vi "FTP Move_Status_Errors.vi"(6 "remote port (21)":u16=21, 8 "error in (no error)":errorcluster, 9 "Dir of file to FTP":path, 10 "FTP input cluster":T1 {"FTP Timeout (S)" min=0 max=300 step=1}, 11 "File to Move":string) -> (1 "concatenated string of Error":string, 3 "FTP completed (true = good)":bool)   [LabVIEW 2011]
uses:
  Controls/FTP Credintials.ctl
  <vilib>/addons/internet/NI_InternetTK_FTP_VIs.lvlib
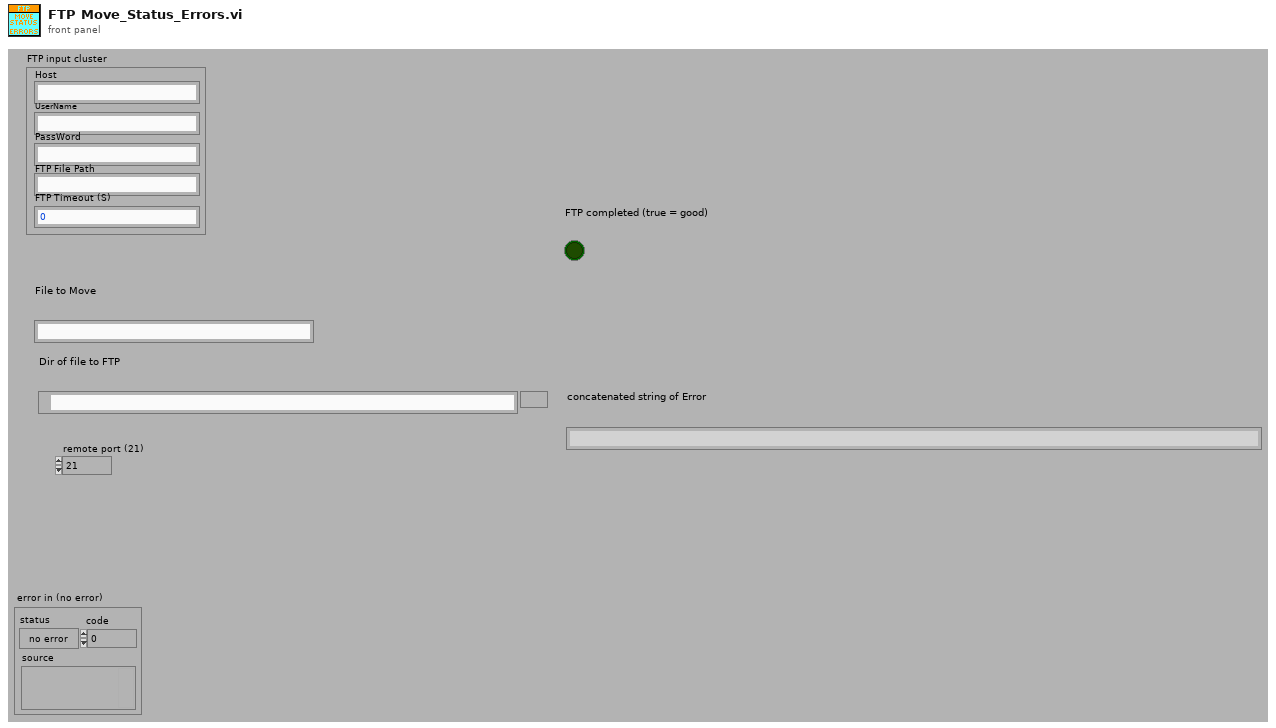
[diagram p1: front panel]
types:
  T1 = typedef "FTP Credintials.ctl" = cluster{"Host":string, "UserName":string, "PassWord":string, "FTP File Path":string, "FTP Timeout (S)":i32, "Active or Passive":bool, "ASCII or Binary":bool}
  T2 = typedef "FTP Session.ctl" = refnum<k1>
  T3 = cluster{string, "appended path":path, "ASCII or Binary":bool, string}
  T4 = cluster{string, "appended path":path, "ASCII or Binary":bool, string}[]
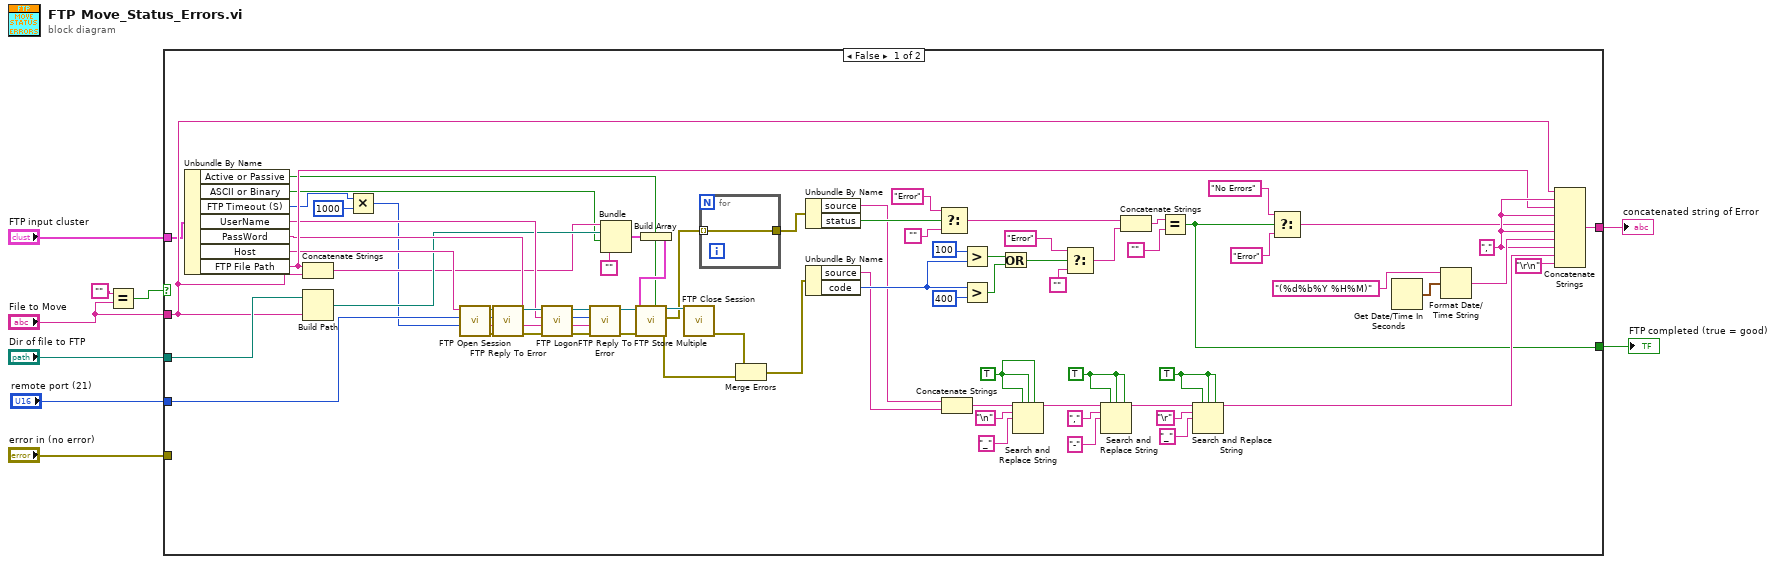
[diagram p0: block diagram]
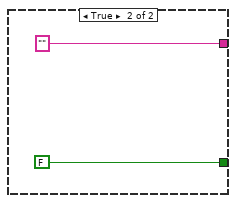
[diagram p2: hidden frame]
diagram:
  n1 = Equal?(x="", y="File to Move") -> (x = y?=w3:bool)
  n2 = case shown="False" w3 {
    tunnel: "Dir of file to FTP" -> [w69 _]
    tunnel: [w68 ""] -> w8
    tunnel: "File to Move" -> [w67 _]
    tunnel: "FTP input cluster" -> [w66 _]
    tunnel: [w12 FALSE] -> w7
    tunnel: "error in (no error)" -> [_ _]
    tunnel: "remote port (21)" -> [w29 _]
    frame False {
      w61 = TRUE ("replace all? (F)")
      w60 = TRUE ("replace all? (F)")
      w51 = TRUE ("replace all? (F)")
      w71 = "," ("string")
      n3 = Unbundle By Name(w66) -> ("Active or Passive"=w10:bool, "ASCII or Binary"=w11:bool, "FTP Timeout (S)"=w21:i32, "UserName"=w32:string, "PassWord"=w33:string, "Host"=w34:string, "FTP File Path"=w70:string)
      n4 = Concatenate Strings(w70, w67) -> (w30:string)
      n5 = Build Path(base path=w69, name or relative path=w67) -> (appended path=w31:path)
      n6 = Multiply(x=w21, y=1000) -> (x*y=w22:i32)
      n7 = call <vilib>:"FTP Open Session.vi"("timeout ms (60000)"=w22, "remote port (21)"=w29, "address"=w34) -> ("error out"=w26:errorcluster, "reply string"=w40:string, "reply code"=w39:i32, "ftp session"=w38:T2)  [unwired: 1 in, 4 out]
      n8 = call <vilib>:"FTP Reply To Error.vi"("error in (no error)"=w26, "reply string in"=w40, "reply code in"=w39, "ftp session"=w38) -> ("error out"=w42:errorcluster, "ftp session out"=w41:T2)  [unwired: 2 out]
      n9 = call <vilib>:"FTP Logon.vi"("error in (no error)"=w42, "password"=w33, "user"=w32, "ftp session"=w41) -> ("error out"=w43:errorcluster, "reply string"=w46:string, "reply code"=w45:i32, "ftp session out"=w44:T2)  [unwired: 4 out]
      n10 = call <vilib>:"FTP Reply To Error.vi"("error in (no error)"=w43, "reply string in"=w46, "reply code in"=w45, "ftp session"=w44) -> ("error out"=w47:errorcluster, "ftp session out"=w48:T2)  [unwired: 2 out]
      n11 = Bundle(w30, "appended path"=w31, "ASCII or Binary"=w11, "") -> (w36:T3)  [unwired: 1 out]
      n12 = Build Array(w36) -> (w35:T4)
      n13 = call <vilib>:"FTP Store Multiple.vi"("active (T)"=w10, "error in (no error)"=w47, "file specifications"=w35, "ftp session"=w48) -> ("error out"=w24:errorcluster, "file errors"=w28:errorcluster[], "ftp session out"=w49:T2)  [unwired: 5 out]
      n14 = call <vilib>:"FTP Close Session.vi"("ftp session"=w49) -> ("error out"=w25:errorcluster)  [unwired: 1 in, 9 out]
      n15 = for {
        tunnel: w28 -> [w86] mode=indexing
        tunnel: [w86] -> w27
      }
      n16 = Merge Errors(w25, w24) -> (w23:errorcluster)
      n17 = Unbundle By Name(w27) -> ("source"=w16:string, "status"=w65:bool)
      n18 = Unbundle By Name(w23) -> ("source"=w15:string, "code"=w75:i32)
      n19 = Select(t="Error", s=w65, f="") -> (s? t:f=w80:string)
      n20 = Concatenate Strings(w16, w15) -> (w17:string)
      n21 = Greater?(x=100, y=w75) -> (0:w73:bool)
      n22 = Greater?(x=w75, y=400 ("x")) -> (0:w76:bool)
      n23 = Or(x=w73, y=w76) -> (x .or. y?=w64:bool)
      n24 = Search and Replace String(replace all?=w51, case sensitive?=w51, multiline?=w51, input string=w17, search string="\n", replace string="_" ("replace string (\"\")")) -> (result string=w56:string)  [unwired: 2 in, 3 out]
      n25 = Select(t="Error", s=w64, f="") -> (s? t:f=w81:string)
      n26 = Search and Replace String(replace all?=w60, case sensitive?=w60, multiline?=w60, input string=w56, search string=",", replace string="-" ("replace string (\"\")")) -> (result string=w59:string)  [unwired: 2 in, 3 out]
      n27 = Concatenate Strings(w80, w81) -> (w78:string)
      n28 = Equal?(x=w78, y="") -> (x = y?=w12:bool)
      n29 = Search and Replace String(replace all?=w61, case sensitive?=w61, multiline?=w61, input string=w59, search string="\r", replace string="_" ("replace string (\"\")")) -> (result string=w50:string)  [unwired: 2 in, 3 out]
      n30 = Select(t="No Errors", s=w12, f="Error" ("t")) -> (s? t:f=w14:string)
      n31 = Get Date/Time In Seconds() -> (seconds since 1Jan1904=w85:timestamp)
      n32 = Format Date/Time String(time format string (%c)="(%d%b%Y %H%M)", seconds (now)=w85) -> (date/time string=w83:string)  [unwired: 1 in]
      n33 = Concatenate Strings(w67, w71, w70, w71, w14, w71, w83, w71, w50, "\r\n") -> (w68:string)
    }
    frame True {
    }
  }
  "concatenated string of Error" <- w8
  "FTP completed (true = good)" <- w7
